vi "Broadcast Leaf Notifiers.vi"(8 "error in (no error)":errorcluster, 10 "Notification":i64, 11 "Root Actor in":refnum<class "Root Actor.lvclass">) -> (0 "error out":errorcluster, 3 "Root Actor out":refnum<class "Root Actor.lvclass">)   [LabVIEW 2024, in "Root Actor.lvclass"]
uses:
  Root Actor.lvclass
  Root Actor.lvclass/Root Actor.ctl
  Notifier/Notifier.lvclass
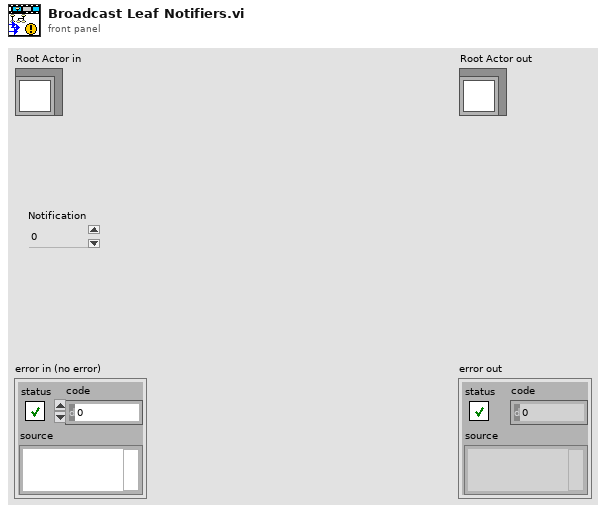
[diagram p1: front panel]
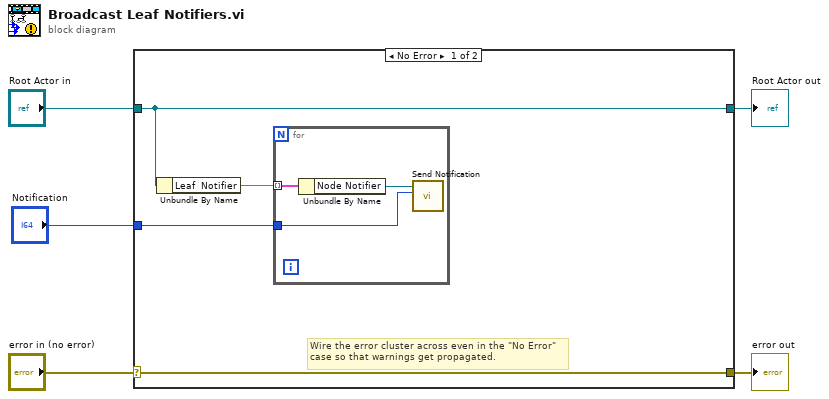
[diagram p0: block diagram]
diagram:
  n1 = case shown="No Error" "error in (no error)" {
    selector: "error in (no error)" -> [w9 w14]
    tunnel: [w9 w14] -> w4
    tunnel: [w8 w13] -> w2
    tunnel: "Root Actor in" -> [w8 w13]
    tunnel: "Notification" -> [w6 _]
    frame No Error {
      # "Wire the error cluster across even in the \"No Error\"\ncase so that warnings get propagated."
      n2 = Unbundle By Name(w8) -> ("Leaf  Notifier"=w7:map{i64[], refnum<class "Notifier.lvclass">})
      n3 = for {
        tunnel: w7 -> [w12] mode=indexing
        tunnel: w6 -> [w10]
        n4 = Unbundle By Name(w12) -> ("Node Notifier"=w11:refnum<class "Notifier.lvclass">)
        n5 = call-dynamic "Send Notification.vi"("Notification"=w10, "Notifier in"=w11) -> ()  [unwired: 7 in, 3 out]
      }
    }
    frame Error {
    }
  }
  "error out" <- w4
  "Root Actor out" <- w2
